vi "Write Cmd and Wait.vi"(8 "error in (no error)":errorcluster, 9 "Message Data":variant, 10 "User Event in":refnum<user-event>, 11 "Data Cluster":T1) -> (0 "error out":errorcluster, 2 "Return Payload":string, 5 "Command":string)   [LabVIEW 2017, in "SSH.lvlib"]
doc: "Sends out a command and waits for the response back - actions the \"Write Command\" request"
uses:
  SSH.lvlib
  Return Request Configuration.ctl
  Response Configuration.ctl
  Module Data--cluster.ctl
  C:/Users/ukhornp/Documents/SSH/References/Renci.SshNet.dll
  References/Renci.SshNet.dll
  Write Command Argument--cluster.ctl
  Write Command (Reply Payload)--cluster.ctl
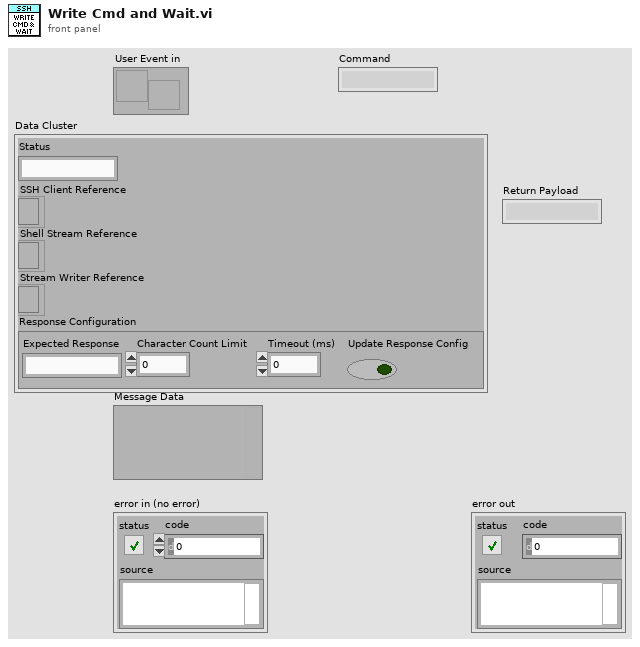
[diagram p1: front panel]
types:
  T1 = typedef "SSH.lvlib/Module Data--cluster.ctl" = cluster{"Status":string, "SSH Client Reference":refnum<k24>, "Shell Stream Reference":refnum<k24>, "Stream Writer Reference":refnum<k24>, "Response Configuration":T2}
  T2 = typedef "SSH.lvlib/Response Configuration.ctl" = cluster{"Expected Response":string, "Character Count Limit":i32, "Timeout (ms)":u32, "Update Response Config":bool}
  T3 = typedef "SSH.lvlib/Return Request Configuration.ctl" = cluster{"Response Configuration":T2, "Return Notifier":refnum<notifier>, "Response Requested":bool, "Command":string, "Initial Timer Value":u32}
  T4 = typedef "SSH.lvlib/Write Command (Reply Payload)--cluster.ctl" = cluster{"Write Command_error":errorcluster, "Return String Payload":string}
  T5 = typedef "SSH.lvlib/Write Command Argument--cluster.ctl" = cluster{"Module ID":i32, "Command":string, "Wait Notifier":refnum<notifier>, "wait for reply":bool}
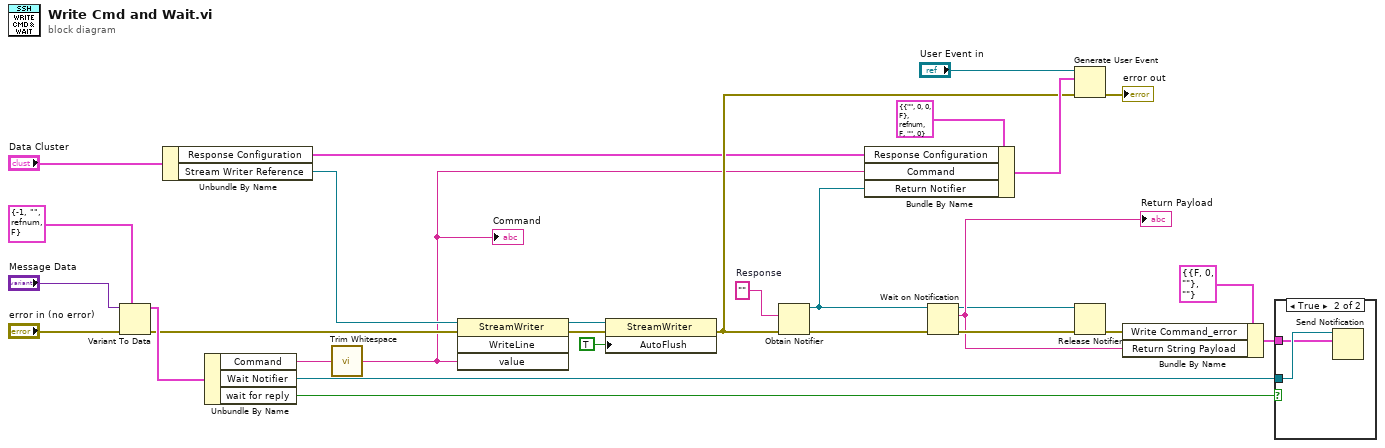
[diagram p0: block diagram]
diagram:
  w15 = ""  # Response
  n1 = Variant To Data(error in="error in (no error)", type=T5 {"Module ID"=-1, "Command"="", "Wait Notifier"=refnum, "wait for reply"=FALSE} ("Write Command Argument"), Variant="Message Data") -> (data=w24:T5, error out=w16:errorcluster)
  n2 = Unbundle By Name("Data Cluster") -> ("Response Configuration"=w4:T2, "Stream Writer Reference"=w18:refnum<k24>)
  n3 = Unbundle By Name(w24) -> ("Command"=w2:string, "Wait Notifier"=w25:refnum<notifier>, "wait for reply"=w26:bool)
  n4 = call <vilib>:"Trim Whitespace.vi"("string"=w2) -> ("trimmed string"=w1:string)  [unwired: 1 in]
  "Command" <- w1
  n5 = invoke class="StreamWriter" method="WriteLine"(reference=w18, error in=w16, "value"=w1) -> (reference out=w17:refnum<k24>, error out=w20:errorcluster)  [unwired: 1 in, 2 out]
  n6 = property class="StreamWriter"(reference=w17, error in=w20, "AutoFlush"=TRUE) -> (error out=w6:errorcluster)  [unwired: 1 out]
  n7 = Obtain Notifier(notification data type=w15, error in (no error)=w6) -> (notifier out=w3:refnum<notifier>, error out=w9:errorcluster)  [unwired: 2 in, 1 out]
  n8 = Bundle By Name(cluster=T3 {"Response Configuration"={"Expected Response"="", "Character Count Limit"=0, "Timeout (ms)"=0, "Update Response Config"=FALSE}, "Return Notifier"=refnum, "Response Requested"=FALSE, "Command"="", "Initial Timer Value"=0} ("Return Request"), "Response Configuration"=w4, "Command"=w1, "Return Notifier"=w3) -> (w12:T3)
  n9 = Wait on Notification(notifier=w3, error in (no error)=w9) -> (notifier out=w7:refnum<notifier>, notification=w10:string, error out=w11:errorcluster)  [unwired: 2 in, 1 out]
  "Return Payload" <- w10
  n10 = Generate User Event(user event="User Event in", event data cluster=w12, error in=w6) -> (error out=→"error out":errorcluster)  [unwired: 1 in, 1 out]
  n11 = Release Notifier(notifier=w7, error in (no error)=w11) -> (error out=w8:errorcluster)  [unwired: 1 in, 2 out]
  n12 = Bundle By Name(cluster=T4 {"Write Command_error"={"status"=FALSE, "code"=0, "source"=""}, "Return String Payload"=""} ("Write Command (Reply Payload)"), "Write Command_error"=w8, "Return String Payload"=w10) -> (w27:T4)
  n13 = case shown="True" w26 {
    tunnel: w25 -> [_ w31]
    tunnel: w27 -> [_ w30]
    frame False {
    }
    frame True {
      n14 = Send Notification(notification=w30, notifier=w31) -> ()  [unwired: 1 in, 2 out]
    }
  }
